vi "Write Force Demand.vi"(10 "Force Demand":T1 format="%.6f", 11 "ForceDemand in":refnum<class "ForceDemand.lvclass">) -> (3 "ForceDemand out":refnum<class "ForceDemand.lvclass">)   [LabVIEW 2013, in "ForceDemand.lvclass"]
uses:
  ForceDemand.lvclass
  Typedefs/ForceDemand.ctl
  ForceDemand.lvclass/ForceDemand.ctl
  Typedefs/M2AADTTypedefs.lvlib
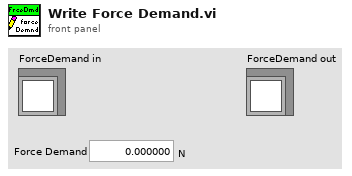
[diagram p1: front panel]
types:
  T1 = typedef "M2AADTTypedefs.lvlib/ForceDemand.ctl" = dbl[unit]
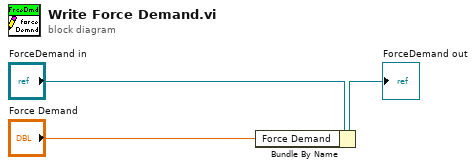
[diagram p0: block diagram]
diagram:
  n1 = Bundle By Name(cluster="ForceDemand in", "Force Demand"="Force Demand") -> (→"ForceDemand out":refnum<class "ForceDemand.lvclass">)
